vi "Read datatype.vi"(8 "error in (no error)":errorcluster, 11 "BooleanPointer in":refnum<class "BooleanPointer.lvclass">) -> (0 "error out":errorcluster, 2 "datatype":string, 3 "BooleanPointer out":refnum<class "BooleanPointer.lvclass">)   [LabVIEW 2014, in "BooleanPointer.lvclass"]
uses:
  BooleanPointer.lvclass
  BooleanPointer.lvclass/BooleanPointer.ctl
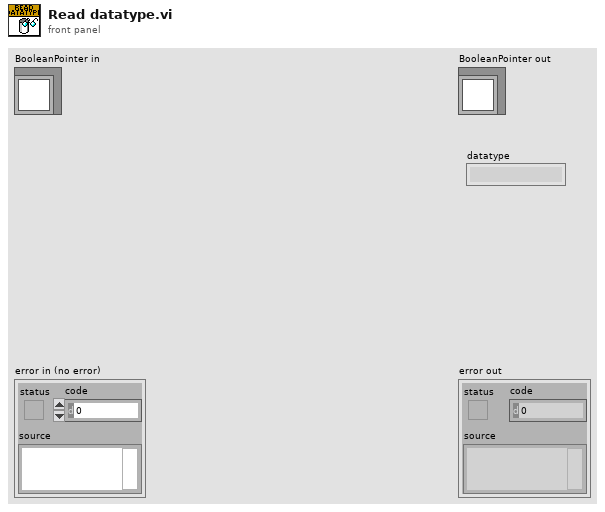
[diagram p1: front panel]
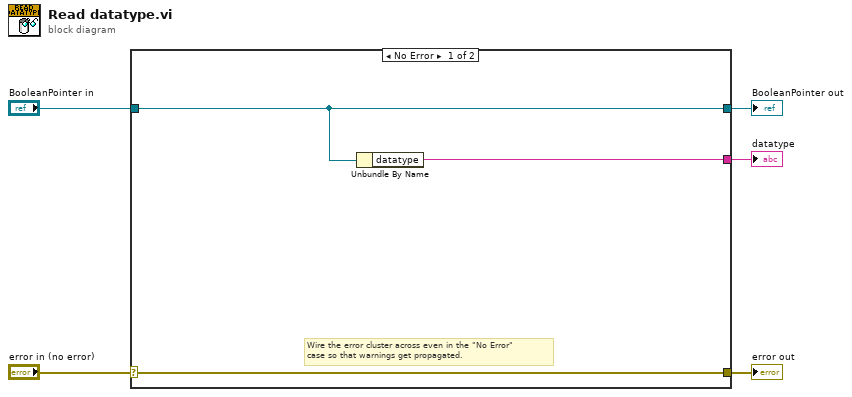
[diagram p0: block diagram]
diagram:
  n1 = case shown="No Error" "error in (no error)" {
    selector: "error in (no error)" -> [w8 w10]
    tunnel: [w8 w10] -> w4
    tunnel: [w7 w9] -> w2
    tunnel: "BooleanPointer in" -> [w7 w9]
    tunnel: [w6 _] -> w1
    frame No Error {
      # "Wire the error cluster across even in the \"No Error\"\ncase so that warnings get propagated."
      n2 = Unbundle By Name(w7) -> ("datatype"=w6:string)
    }
    frame Error {
    }
  }
  "error out" <- w4
  "BooleanPointer out" <- w2
  "datatype" <- w1
